vi "calibrate.vi"(6 "button":bool, 11 "AI":dbl) -> (3 "scaled AI":dbl)   [LabVIEW 2014]
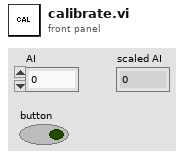
[diagram p1: front panel]
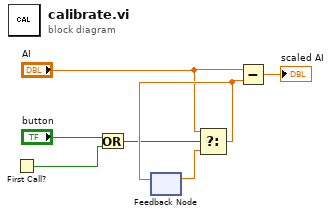
[diagram p0: block diagram]
diagram:
  n1 = First Call?() -> (First Call?: T/F=w3:bool)
  n2 = Or(x="button", y=w3) -> (x .or. y?=w5:bool)
  n3 = feedback #1() -> (w1:dbl)  [unwired: 1 in]
  n4 = Select(t="AI", s=w5, f=w1) -> (s? t:f=w6:dbl)
  n5 = feedback-in #1(w6) -> ()
  n6 = Subtract(x="AI", y=w6) -> (x-y=→"scaled AI":dbl)
